vi "Downsample DAQ Data.vi"() -> ()   [LabVIEW 2013]
uses:
  <vilib>/Utility/error.llb/DialogType.ctl
  <vilib>/DAQmx/miscellaneous.llb/DAQmx Fill In Error Info.vi
  <vilib>/Waveform/WDTOps.llb/WDT Append Waveforms DBL.vi
  <vilib>/Analysis/baseanly.llb/Mean (DBL).vi
  <vilib>/DAQmx/read.llb/DAQmx Read (Analog Wfm 1Chan NSamp).vi
  <vilib>/DAQmx/configure/timing.llb/DAQmx Timing (Sample Clock).vi
  <vilib>/DAQmx/create/channels.llb/DAQmx Create Channel (AI-Voltage-Basic).vi
  <resource>/objmgr/daqmx.rc
  <vilib>/Analysis/NI_AALBase.lvlib
panel:
  in  "Downsampling Method":i32(ring) items=["Average", "First Point", "Last Point"]
  out "Time Between Samples (s)":dbl=1000.0 format="%0.2f"
  out "Read Rate (S/s)":dbl=1000.0 format="%0.2f"
  in  "Stop":bool
  out "Waveform Graph":waveform(dbl)[](graph)
  in  "Samples to Read":i32=1000
  in  "Sample Rate (S/s)":dbl=10000.0
  in  "Sample Clock Source":tag="OnboardClock"
  in  "Terminal Configuration":i32(ring)=-1 items=["default"=-1, "RSE"=10083, "NRSE"=10078, "Differential"=10106, "Pseudodifferential"=12529]
  in  "Max Voltage":dbl=5.0
  in  "Min Voltage":dbl=-5.0
  in  "Physical Channel":tag="Dev1/ai0"
  out "Actual Sample Rate":dbl=1000.0 format="%0.2f"
  # "Channel Settings"
  # "Acquired Data"
  # "Timing Settings"
  # "1. Select the channel, bounds, and terminal configuration under \"Channel Settings\"\n\n2. Choose the sampling rate, number of samples to read, and downsampling\n    method under \"Timing Settings\"\n\n3. Run and observe the differences between the raw data and downsampled data"
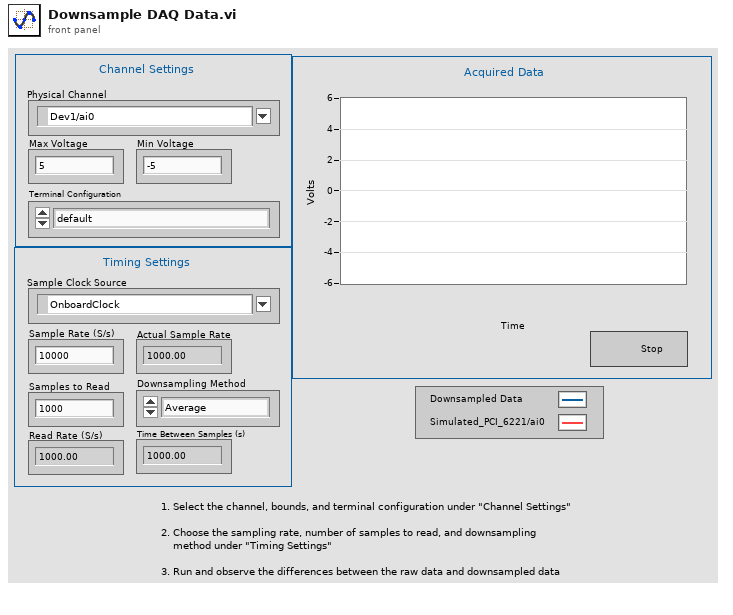
[diagram p1: front panel]
types:
  T1 = typedef "DialogType.ctl" = u16
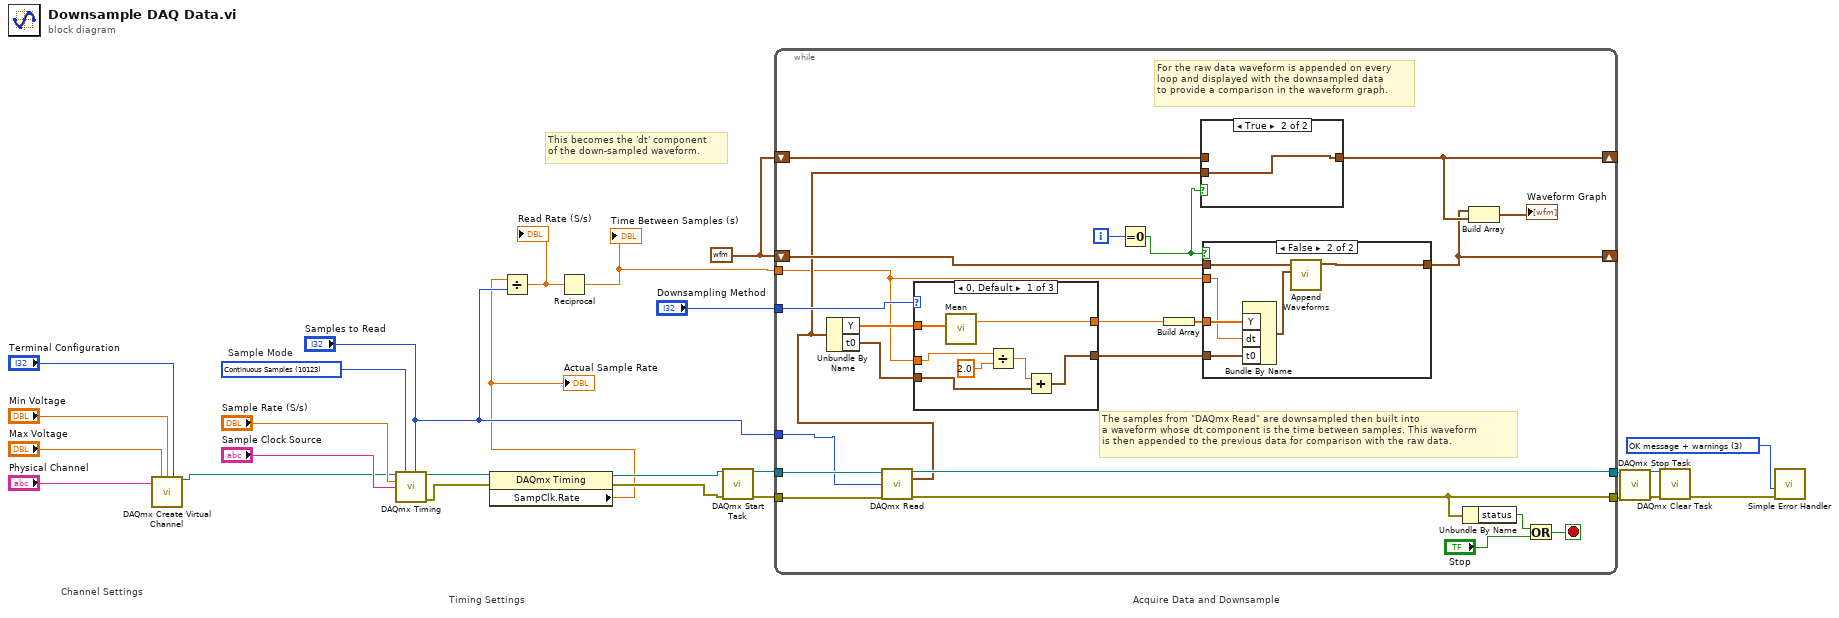
[diagram p0: block diagram]
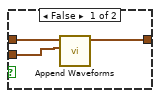
[diagram p2: hidden frame]
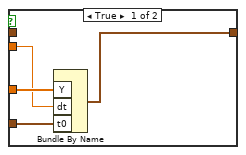
[diagram p3: hidden frame]
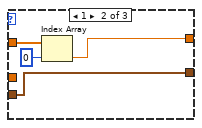
[diagram p4: hidden frame]
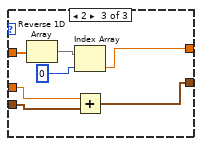
[diagram p5: hidden frame]
diagram:
  w1 = waveform(dbl) {"t0"=timestamp(3364135200 s since 1904-01-01), "dt"=1.0, "Y"=[]}
  w10 = T1 3 items=["no dialog", "OK message", "continue or stop message", "OK message + warnings", "continue/stop + warnings"] ("type of dialog (OK msg:1)")
  w24 = 10123 items=["Finite Samples"=10178, "Continuous Samples"=10123, "Hardware Timed Single Point"=12522]  # Sample Mode
  # "This becomes the 'dt' component\nof the down-sampled waveform."
  # "Acquire Data and Downsample"
  # "Timing Settings"
  # "Channel Settings"
  n1 = call-poly <vilib>:"DAQmx Create Virtual Channel.vi"("maximum value"="Max Voltage", "minimum value"="Min Voltage", "input terminal configuration"="Terminal Configuration", "physical channels"="Physical Channel") -> ("task out"=w7:refnum<k21>)  [unwired: 10 in, 1 out]
  n2 = call-poly <vilib>:"DAQmx Timing.vi"("task/channels in"=w7, "sample mode"=w24, "samples per channel"="Samples to Read", "rate"="Sample Rate (S/s)", "source"="Sample Clock Source") -> ("task out"=w26:refnum<k21>, "error out"=w25:errorcluster)  [unwired: 9 in]
  n3 = property class="DAQmx Timing"(reference=w26, error in=w25) -> (reference out=w9:refnum<k21>, error out=w8:errorcluster, "SampClk.Rate"=w4:dbl)
  "Actual Sample Rate" <- w4
  n4 = Divide(x=w4, y="Samples to Read") -> (x/y=w5:dbl)
  "Read Rate (S/s)" <- w5
  n5 = Reciprocal(x=w5) -> (1/x=w2:dbl)
  "Time Between Samples (s)" <- w2
  n6 = call <vilib>:"DAQmx Start Task.vi"("task/channels in"=w9, "error in"=w8) -> ("task out"=w23:refnum<k21>, "error out"=w22:errorcluster)  [unwired: 12 in]
  n7 = while {
    tunnel: w23 -> [w49]
    tunnel: w22 -> [w48]
    tunnel: [w47] -> w14
    tunnel: [w43] -> w13
    tunnel: "Samples to Read" -> [w42]
    tunnel: "Downsampling Method" -> [w40]
    tunnel: w2 -> [w32]
    shift-right: [w28] -> _
    shift-left: w1 -> [w36]
    shift-right: [w29] -> _
    shift-left: w1 -> [w33]
    i -> [w39]
    stop <- w44 stop-if-true
    # "The samples from \"DAQmx Read\" are downsampled then built into\na waveform whose dt component is the time between samples. This waveform\nis then appended to the previous data for comparison with the raw data."
    # "For the raw data waveform is appended on every\nloop and displayed with the downsampled data\nto provide a comparison in the waveform graph."
    n8 = call-poly <vilib>:"DAQmx Read.vi"("task/channels in"=w49, "number of samples per channel"=w42, "error in"=w48) -> ("task out"=w47:refnum<k21>, "data"=w34:waveform(dbl), "error out"=w43:errorcluster)  [unwired: 10 in]
    n9 = Unbundle By Name(w34) -> ("Y"=w41:dbl[], "t0"=w31:timestamp)
    n10 = case shown="0, Default" w40 {
      tunnel: w41 -> [w70 w74 w78]
      tunnel: [w69 w72 w80] -> w38
      tunnel: w32 -> [w66 _ w76]
      tunnel: w31 -> [w68 w71 w77]
      tunnel: [w67 w71 w75] -> w30
      frame 0, Default {
        n11 = call-poly <vilib>:"Mean.vi"("X"=w70) -> ("mean"=w69:dbl)  [unwired: 1 out]
        n12 = Divide(x=w66, y=2.0) -> (x/y=w65:dbl)
        n13 = Add(x=w65, y=w68) -> (x+y=w67:timestamp)
      }
      frame 1 {
        n14 = Index Array(array=w74, index=0) -> (element=w72:dbl)
      }
      frame 2 {
        n15 = Reverse 1D Array(array=w78) -> (reversed array=w79:dbl[])
        n16 = Index Array(array=w79, index=0) -> (element=w80:dbl)
        n17 = Add(x=w76, y=w77) -> (x+y=w75:timestamp)
      }
    }
    n18 = Equal To 0?(x=w39) -> (x = 0?=w35:bool)
    n19 = Build Array(w38) -> (w37:dbl[])
    n20 = case shown="True" w35 {
      tunnel: w34 -> [w52 w53]
      tunnel: w33 -> [w50 _]
      tunnel: [w51 w53] -> w29
      frame False {
        n21 = call-poly <vilib>:"Append Waveforms.vi"("waveform B"=w52, "waveform A"=w50) -> ("waveform out"=w51:waveform(dbl))  [unwired: 8 in, 1 out]
      }
      frame True {
      }
    }
    n22 = case shown="False" w35 {
      tunnel: w37 -> [w57 w63]
      tunnel: [w56 w62] -> w28
      tunnel: w32 -> [w55 w59]
      tunnel: w36 -> [_ w60]
      tunnel: w30 -> [w54 w58]
      frame True {
        n23 = Bundle By Name("Y"=w57, "dt"=w55, "t0"=w54) -> (w56:waveform(dbl))  [unwired: 1 in]
      }
      frame False {
        n24 = Bundle By Name("Y"=w63, "dt"=w59, "t0"=w58) -> (w61:waveform(dbl))  [unwired: 1 in]
        n25 = call-poly <vilib>:"Append Waveforms.vi"("waveform B"=w61, "waveform A"=w60) -> ("waveform out"=w62:waveform(dbl))  [unwired: 8 in, 1 out]
      }
    }
    n26 = Unbundle By Name(w43) -> ("status"=w45:bool)
    n27 = Build Array(w28, w29) -> (→"Waveform Graph":waveform(dbl)[])
    n28 = Or(x=w45, y="Stop") -> (x .or. y?=w44:bool)
  }
  n29 = call <vilib>:"DAQmx Stop Task.vi"("task/channels in"=w14, "error in"=w13) -> ("task out"=w11:refnum<k21>, "error out"=w12:errorcluster)  [unwired: 12 in]
  n30 = call <vilib>:"DAQmx Clear Task.vi"("task in"=w11, "error in"=w12) -> ("error out"=w21:errorcluster)  [unwired: 13 in]
  n31 = call <vilib>:"Simple Error Handler.vi"("type of dialog (OK msg:1)"=w10, "error in (no error)"=w21) -> ()  [unwired: 3 in, 5 out]
